vi "SPC_get_stream_buffer_size.vi"(6 "Stream Handle":i16, 8 "Error In":errorcluster, 9 "Buffer No":u16, 11 "DLL Path":path) -> (0 "Error Out":errorcluster, 1 "Buffer Size":u32, 3 "DLL Path":path)   [LabVIEW 2017]
doc: "Before calling SPC_get_buffer_from_stream user must know the buffer size and should allocate big enough data buffer.\nThe SPC_get_stream_buffer_size procedure is used to get size of stream's internal buffer number 'buf_no'. \nStream is defined by handle 'stream_hndl'. The procedure works only with 'buffered' streams.\nCall SPC_get_phot_stream_info to get info about current number of stream buffers (field no_of_buf of PhotStreamInfo structure).\n\ninfo@becker-hickl.com"
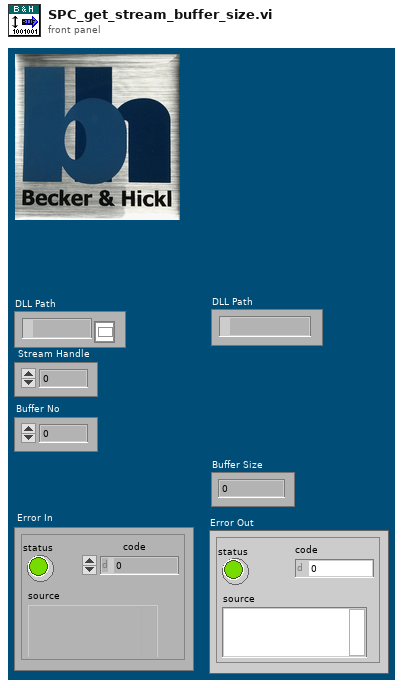
[diagram p1: front panel]
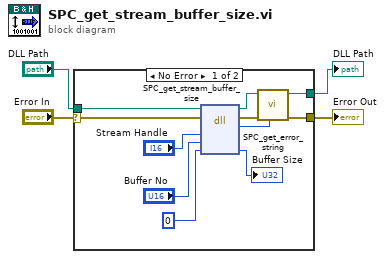
[diagram p0: block diagram]
diagram:
  n1 = case shown="No Error" "Error In" {
    selector: "Error In" -> [w12 w16]
    tunnel: [w10 w16] -> w3
    tunnel: "DLL Path" -> [w9 w17]
    tunnel: [w6 w17] -> w1
    frame No Error {
      n2 = dll-call lib="D:/spcm/lib/lab_view/lv10.0/spcm32.dll" fn="SPC_get_stream_buffer_size"(path in=w9, error in=w12, "stream_hndl"="Stream Handle", "buf_no"="Buffer No", "buf_size"=u32 0 ("Buffer Size")) -> (path out=w7:path, error out=w11:errorcluster, "return type"=w5:i16, "buf_size"=→"Buffer Size":u32)  [unwired: 3 in]
      n3 = call "SPC_get_error_string.vi"("ErrorID"=w5, "Error In"=w11, "DLL Path"=w7) -> ("Error Out"=w10:errorcluster, "DLL Path"=w6:path)  [unwired: 6 in, 1 out]
    }
    frame Error {
    }
  }
  "Error Out" <- w3
  "DLL Path" <- w1
